vi "Varient_Current_Status.vi"(7 "Enum":enum16{"Write", "Read"}(ring), 8 "error in":errorcluster, 11 "Varient Number in":i32) -> (0 "error out":errorcluster, 1 "Batch Size":i32, 2 "Varient Number":i32, 3 "Varient Name":string)   [LabVIEW 2017]
uses:
  <vilib>/Utility/config.llb/Write Key (I32).vi
  <vilib>/Utility/config.llb/Read Key (I32).vi
  <vilib>/Utility/config.llb/NI_LVConfig.lvlib
panel:
  # "Varient Current Status & Count"
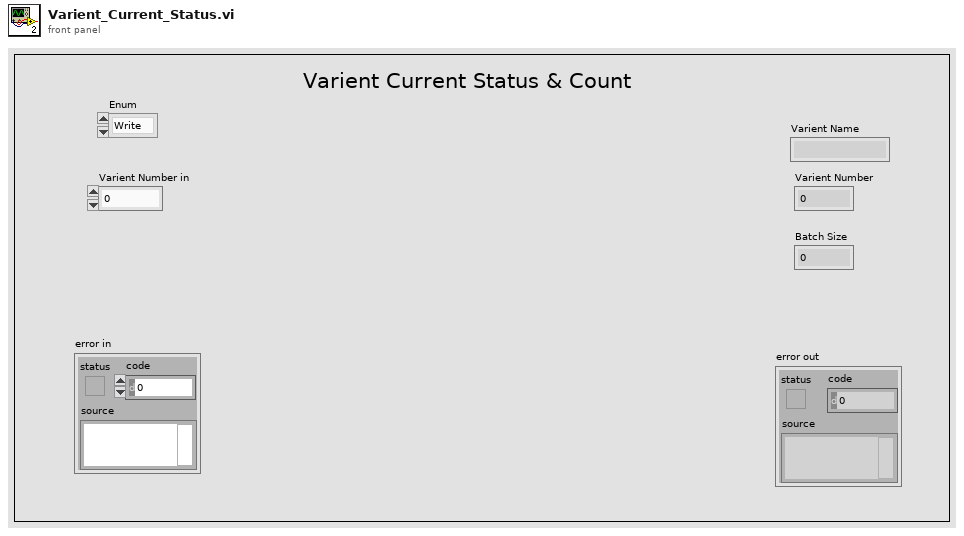
[diagram p1: front panel]
types:
  T1 = enum32{"invalid app kind", "Development System", "Run Time System", "Student Edition", "Embedded LabVIEW", "Evaluation", "Custom"}
  T2 = typedef "NI_LVConfig.lvlib/Config Data RefNum.ctl" = refnum<k1>
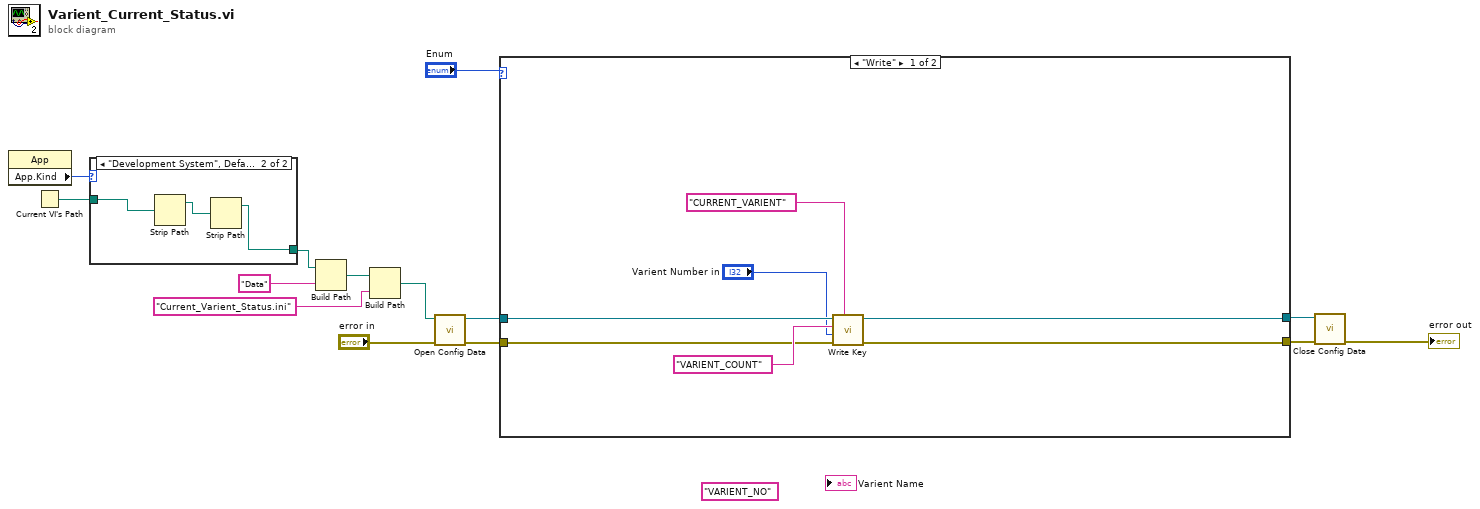
[diagram p0: block diagram]
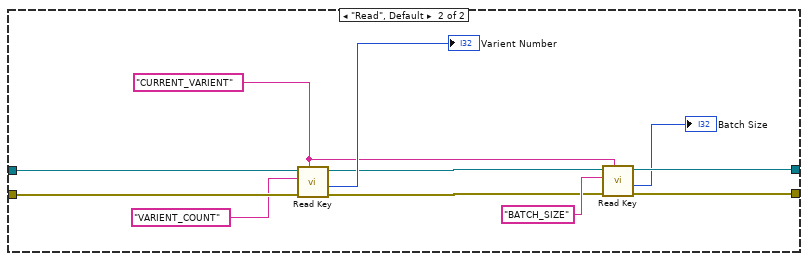
[diagram p2: hidden frame]
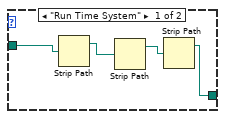
[diagram p3: hidden frame]
diagram:
  (unwired) "VARIENT_NO" ("name or relative path")
  n1 = property class="App"() -> ("App.Kind"=w13:T1)  [unwired: 2 in, 2 out]
  n2 = Current VI's Path() -> (path=w14:path)
  n3 = case shown="\"Development System\", Default" w13 {
    tunnel: w14 -> [w16 w20]
    tunnel: [w15 w19] -> w11
    frame "Run Time System" {
      n4 = Strip Path(path=w16) -> (stripped path=w18:path)  [unwired: 1 out]
      n5 = Strip Path(path=w18) -> (stripped path=w17:path)  [unwired: 1 out]
      n6 = Strip Path(path=w17) -> (stripped path=w15:path)  [unwired: 1 out]
    }
    frame "Development System", Default {
      n7 = Strip Path(path=w20) -> (stripped path=w21:path)  [unwired: 1 out]
      n8 = Strip Path(path=w21) -> (stripped path=w19:path)  [unwired: 1 out]
    }
  }
  n9 = Build Path(base path=w11, name or relative path="Data") -> (appended path=w12:path)
  n10 = Build Path(base path=w12, name or relative path="Current_Varient_Status.ini") -> (appended path=w10:path)
  n11 = call <vilib>:"Open Config Data.vi"("error in (no error)"="error in", "configuration file path"=w10) -> ("error out"=w6:errorcluster, "refnum"=w7:T2)  [unwired: 7 in, 1 out]
  n12 = case shown="\"Write\"" "Enum" {
    tunnel: w7 -> [w24 w39]
    tunnel: w6 -> [w26 w38]
    tunnel: [w25 w34] -> w3
    tunnel: [w23 w32] -> w2
    frame "Write" {
      n13 = call-poly <vilib>:"Write Key.vi"("section"="CURRENT_VARIENT" ("name or relative path"), "error in (no error)"=w26, "value"="Varient Number in", "key"="VARIENT_COUNT" ("name or relative path"), "refnum"=w24) -> ("error out"=w25:errorcluster, "refnum out"=w23:T2)  [unwired: 4 in, 1 out]
    }
    frame "Read", Default {
      w29 = "CURRENT_VARIENT" ("name or relative path")
      n14 = call-poly <vilib>:"Read Key.vi"("section"=w29, "error in (no error)"=w38, "key"="VARIENT_COUNT" ("name or relative path"), "refnum"=w39) -> ("error out"=w35:errorcluster, "value"=→"Varient Number":i32, "refnum out"=w33:T2)  [unwired: 4 in, 1 out]
      n15 = call-poly <vilib>:"Read Key.vi"("section"=w29, "error in (no error)"=w35, "key"="BATCH_SIZE" ("name or relative path"), "refnum"=w33) -> ("error out"=w34:errorcluster, "value"=→"Batch Size":i32, "refnum out"=w32:T2)  [unwired: 4 in, 1 out]
    }
  }
  n16 = call <vilib>:"Close Config Data.vi"("error in (no error)"=w3, "refnum"=w2) -> ("error out"=→"error out":errorcluster)  [unwired: 8 in, 1 out]
